vi "LaunchPythonMethod.vi"(8 "Error In":errorcluster, 9 "Method Name":string, 10 "Python Module Path":path, 11 "Python session":refnum<k35>) -> (0 "Error Out":errorcluster)   [LabVIEW 2019]
panel:
  out "return value":string
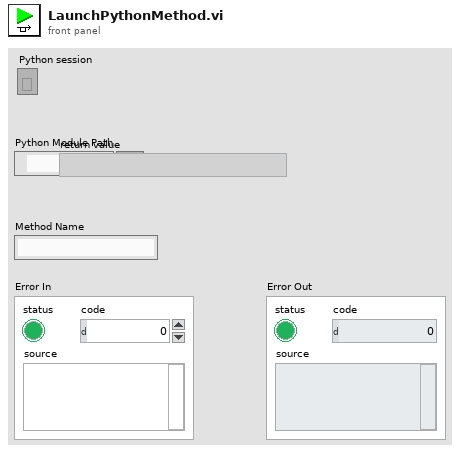
[diagram p1: front panel]
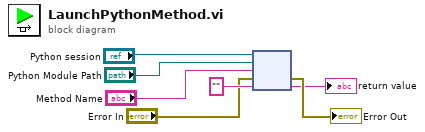
[diagram p0: block diagram]
diagram:
  n1 = node("Python session", "Python Module Path", "Method Name", "Error In", "" ("Python version")) -> (→"Error Out":errorcluster, →"return value":string)  [unwired: 3 out]
